vi "Actor Core.vi"(8 "error in":errorcluster, 11 "ConfigurationLayout in":refnum<class "LeftListboxViewManager.lvclass">=refnum) -> (0 "error out":errorcluster, 3 "Actor out":refnum<class "Actor.lvclass">)   [LabVIEW 2015, in "LeftListboxViewManager.lvlib" / "LeftListboxViewManager.lvclass"]
doc: "(<B>Filename</B>: Actor Framework.lvlib:Actor.lvclass:Actor Core.vi)\n\nReceives messages to the actor, reacts to them, and initiates any error handling that may shut the actor down.\n\nDescendant classes may override this VI to append parallel tasks for the actor to complete while it handles messages. Overrides use the Call Parent Method node.\n\n<License>\nCopyright © 2017 Composed Systems, LLC | All rights reserved\nwww.composed.io\n\nAuthor: Ethan Stern <ethan.stern@composed.io>\n\nThis software is provided \"AS IS\" WITHOUT WARRANTIES, either express or implied, AND IS FOR EDUCATIONAL PURPOSES ONLY.\n</License>"
uses:
  LeftListboxViewManager.lvclass
  <vilib>/ActorFramework/Actor/Actor.lvclass
  LeftListboxViewManager.lvclass/LeftListboxViewManager.ctl
  <vilib>/ActorFramework/Actor/Actor.lvclass/Actor.ctl
  <vilib>/ActorFramework/Message Enqueuer/Message Enqueuer.lvclass/Message Enqueuer.ctl
  LeftListboxViewManager Messages/Set View by Listbox Index Msg/Set View by Listbox Index Msg.lvclass/Set View by Listbox Index Msg.ctl
  <vilib>/ActorFramework/Message Enqueuer/Init from Existing Queue.vi
  <vilib>/ActorFramework/Message Enqueuer/Enqueue.vi
  <vilib>/ActorFramework/Message Priority Queue/Priority Enqueue.vi
  <vilib>/ActorFramework/Message Enqueuer/Message Enqueuer.lvclass
  LeftListboxViewManager Messages/Set View by Listbox Index Msg/Set View by Listbox Index Msg.lvclass
  Framework/IViewManager/IViewManager/IViewManager.lvclass
  Framework/IViewable/ProtectedSubpanel/ProtectedSubpanel.lvclass
panel:
  in  "Listbox":i32(listbox)
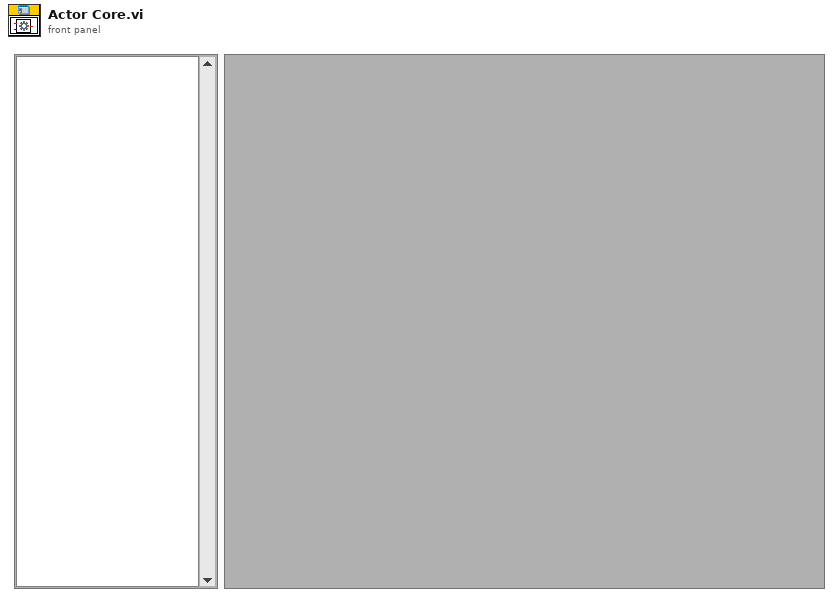
[diagram p1: front panel]
types:
  T1 = typedef "IViewable.lvlib/ProtectedSubpanel.lvclass/Protected Subpanel Reference.ctl" = refnum<data-value>
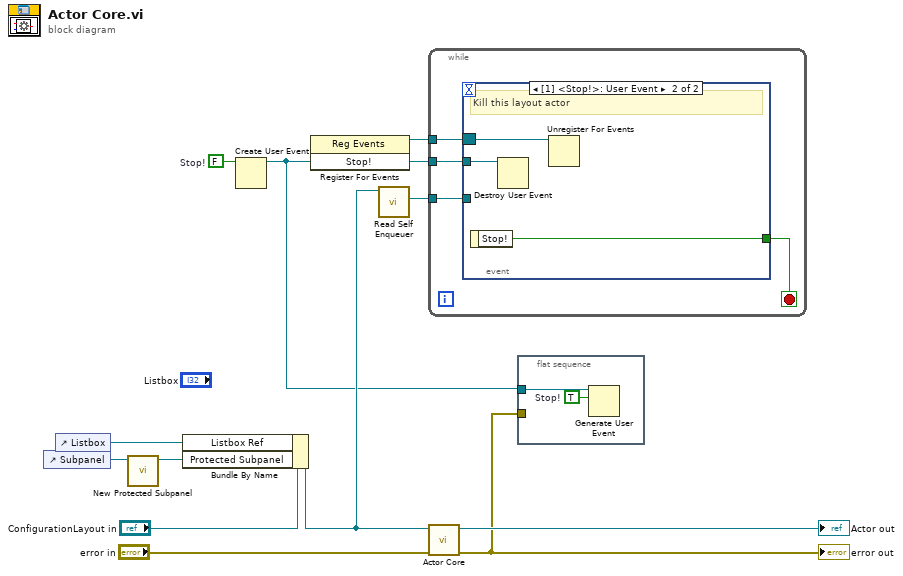
[diagram p0: block diagram]
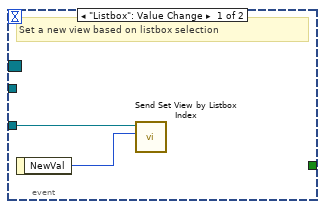
[diagram p2: hidden frame]
diagram:
  w6 = FALSE  # Stop!
  n1 = control-ref of="Subpanel"() -> (w1:refnum<vi>)
  n2 = control-ref of="Listbox"() -> (w9:refnum<vi>)
  n3 = call "New Protected Subpanel.vi"("SubPnl Refnum"=w1) -> ("Protected Subpanel"=w2:T1)  [unwired: 9 in, 1 out]
  n4 = Bundle By Name(cluster="ConfigurationLayout in", "Listbox Ref"=w9, "Protected Subpanel"=w2) -> (w8:refnum<class "LeftListboxViewManager.lvclass">)
  n5 = Create User Event(user event datatype=w6) -> (user event=w4:refnum<user-event>)  [unwired: 1 in, 1 out]
  n6 = register-events(w4) -> (reference out=w5:refnum<event-registration>)  [unwired: 2 in, 1 out]
  n7 = call <vilib>:"Read Self Enqueuer.vi"("Actor"=w8) -> ("Self Enqueuer"=w7:refnum<class "Message Enqueuer.lvclass">)  [unwired: 10 in]
  n8 = while {
    tunnel: w7 -> [w16]
    tunnel: w5 -> [w15]
    tunnel: w4 -> [w13]
    stop <- w14 stop-if-true
    n9 = event shown="[1] <Stop!>: User Event" {
      selector: w15 -> [_ w20]
      dyn-events: _ -> [_ _]
      timeout: _ -> [_ _]
      tunnel: w16 -> [w18 _]
      tunnel: [_ w21] -> w14
      tunnel: w13 -> [_ w19]
      event "Listbox": Value Change {
        # "Set a new view based on listbox selection"
        n10 = event-data() -> ("NewVal"=w17:i32)  [unwired: 1 in]
        n11 = call "Send Set View by Listbox Index.vi"("Index"=w17, "Message Enqueuer"=w18) -> ()  [unwired: 8 in, 2 out]
      }
      event User Event {
        # "Kill this layout actor"
        n12 = event-data() -> ("Stop!"=w21:bool)  [unwired: 1 in]
        n13 = Destroy User Event(user event=w19) -> ()  [unwired: 1 in, 1 out]
        n14 = Unregister For Events(event registration refnum=w20) -> ()  [unwired: 1 in, 1 out]
      }
    }
  }
  n15 = call-parent "Actor Core.vi"("error in"="error in", "IViewable In"=w8) -> ("error out"=w3:errorcluster, "Actor out"=→"Actor out":refnum<class "Actor.lvclass">)  [unwired: 8 in]
  "error out" <- w3
  n16 = flat-sequence {
    tunnel: w4 -> [w22]
    tunnel: w3 -> [_]
    frame #0 {
      w23 = TRUE  # Stop!
      n17 = Generate User Event(user event=w22, event data cluster=w23) -> ()  [unwired: 2 in, 2 out]
    }
  }
